vi "QR_error_generator.vi"(8 "Error In":errorcluster, 11 "CODIGO QR LEÍDO?":bool) -> (0 "Error Out":errorcluster)   [LabVIEW 2019]
uses:
  <vilib>/Utility/error.llb/Error Cluster From Error Code.vi
  <vilib>/ErrorRing/Error Ring.xnode
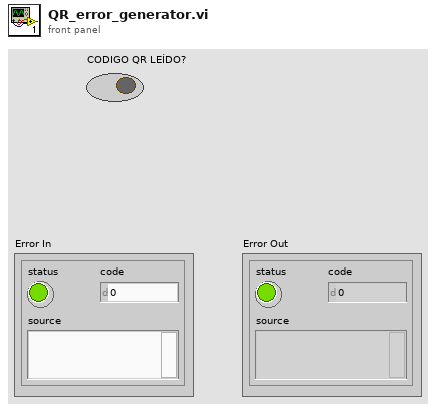
[diagram p1: front panel]
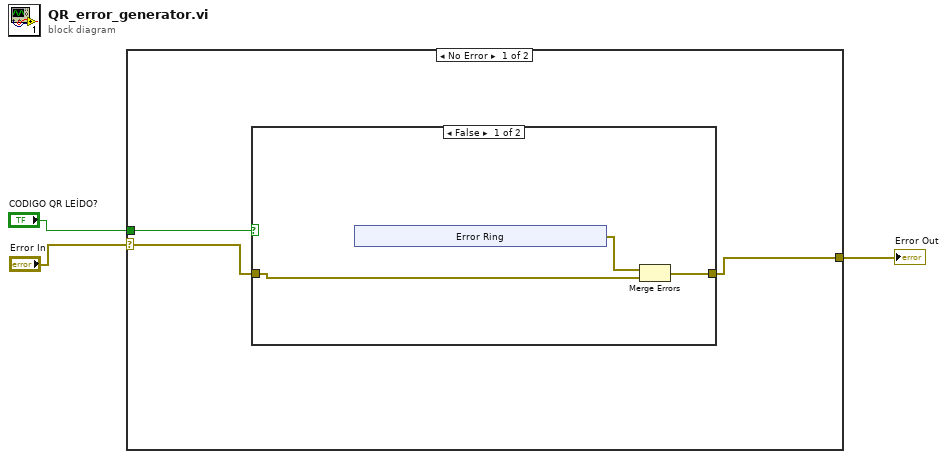
[diagram p0: block diagram]
diagram:
  n1 = case shown="No Error" "Error In" {
    selector: "Error In" -> [w5 w16]
    tunnel: "CODIGO QR LEÍDO?" -> [w6 _]
    tunnel: [w4 w16] -> w1
    frame No Error {
      n2 = case shown="False" w6 {
        tunnel: w5 -> [w9 w15]
        tunnel: [w7 w15] -> w4
        frame False {
          n3 = xnode "Error Ring"() -> ("error out"=w8:errorcluster)
          n4 = Merge Errors(w8, w9) -> (w7:errorcluster)
        }
        frame True {
        }
      }
    }
    frame Error {
    }
  }
  "Error Out" <- w1
